vi "recursively populate local multi-tree ctl.vi"(8 "error in (no error)":errorcluster, 10 "multi-selectable tree ctl ref":refnum<vi>, 11 "Object path":string="IndivITX/Test1/SA03008N.20190801.000000.itx") -> (0 "error out":errorcluster, 2 "multi-selectable tree ctl ref 2":refnum<vi>)   [LabVIEW 2016]
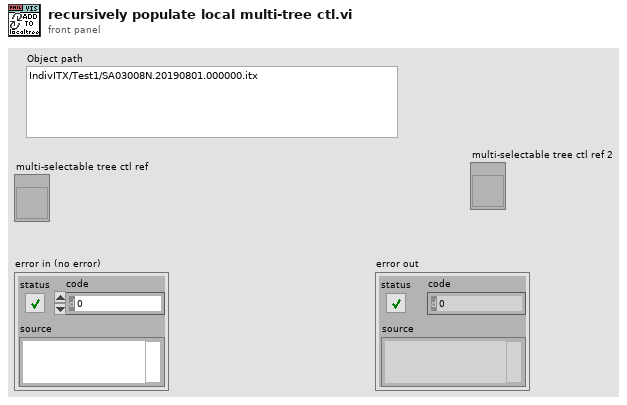
[diagram p1: front panel]
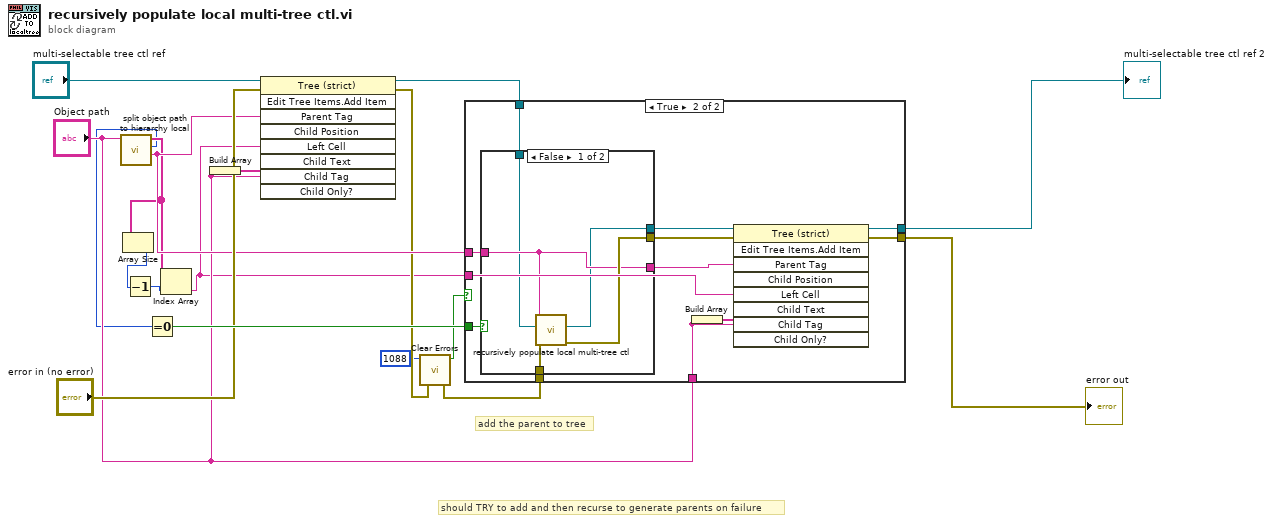
[diagram p0: block diagram]
diagram:
  # "should TRY to add and then recurse to generate parents on failure"
  # "add the parent to tree"
  n1 = call "split object path to hierarchy local.vi"("Object path"="Object path") -> ("parent path"=w15:string, "layers"=w4:i32, "hierarchy"=w7:string[])  [unwired: 8 in]
  n2 = Array Size(array=w7) -> (size(s)=w5:i32)
  n3 = Decrement(x=w5) -> (x-1=w6:i32)
  n4 = Equal To 0?(x=w4) -> (x = 0?=w18:bool)
  n5 = Index Array(array=w7, index=w6) -> (element=w3:string)
  n6 = Build Array("Object path") -> (w14:string[])
  n7 = invoke on="Invoke Node" class="Tree (strict)" method="Edit Tree Items.Add Item"(reference="multi-selectable tree ctl ref", error in="error in (no error)", "Parent Tag"=w15, "Left Cell"=w3, "Child Text"=w14, "Child Tag"="Object path") -> (reference out=w13:refnum<vi>, error out=w11:errorcluster)  [unwired: 3 in, 7 out]
  n8 = call <vilib>:"Clear Errors.vi"("error in (no error)"=w11, "specific error code to clear (0: all)"=1088) -> ("error out"=w16:errorcluster, "specific error cleared?"=w10:bool)  [unwired: 4 in]
  n9 = case shown="True" w10 {
    tunnel: [w19 w25] -> w8
    tunnel: w18 -> [_ w32]
    tunnel: [w20 w26] -> w1
    tunnel: w16 -> [w19 w31]
    tunnel: w15 -> [_ w30]
    tunnel: w13 -> [w20 w29]
    tunnel: "Object path" -> [_ w22]
    tunnel: w3 -> [_ w21]
    frame False {
    }
    frame True {
      n10 = case shown="False" w32 {
        tunnel: w31 -> [w37 w40]
        tunnel: w30 -> [w35 w38]
        tunnel: [w36 w40] -> w28
        tunnel: w29 -> [w33 w39]
        tunnel: [w34 w39] -> w27
        tunnel: [w35 w38] -> w24
        frame False {
          n11 = call "recursively populate local multi-tree ctl.vi"("error in (no error)"=w37, "multi-selectable tree ctl ref"=w33, "Object path"=w35) -> ("error out"=w36:errorcluster, "multi-selectable tree ctl ref 2"=w34:refnum<vi>)  [unwired: 7 in]
        }
        frame True {
        }
      }
      n12 = Build Array(w22) -> (w23:string[])
      n13 = invoke on="Invoke Node" class="Tree (strict)" method="Edit Tree Items.Add Item"(reference=w27, error in=w28, "Parent Tag"=w24, "Left Cell"=w21, "Child Text"=w23, "Child Tag"=w22) -> (reference out=w26:refnum<vi>, error out=w25:errorcluster)  [unwired: 3 in, 7 out]
    }
  }
  "error out" <- w8
  "multi-selectable tree ctl ref 2" <- w1
